vi "Fetch Multiple Record Single Channel (U64).vi"(5 "FIFO Type":enum16{"FPGA to Host FIFO (U64)", "Generic"}(ring), 7 "Timeout (s)":i32=5, 8 "error in":errorcluster, 10 "Records to Fetch":i32, 11 "FPGA VI Reference In":refnum<k20>) -> (0 "error out":errorcluster, 2 "Acquired Data":u64[](array[numeric]), 3 "FPGA VI Reference Out":refnum<k20>, 4 "Elements Remaining":u32)   [LabVIEW 2011]
uses:
  <userlib>/FlexRIO Host Library/FlexRIO Host API/Acquire/Fetch/Fetch Acquired Data (U64).vi
  <vilib>/Utility/error.llb/Error Cluster From Error Code.vi
  <vilib>/rvi/errors/niLvFpgaAdjustHostInterfaceError.vi
  <vilib>/rvi/interface/nirviReadWriteControl/nirviReadWriteControl.xnode
  NiFpgaLv.dll
  <vilib>/rvi/interface/Simulation/niFpgaSimulationCallBeginRW.vi
  <userlib>/FlexRIO Host Library/FlexRIO Host Library (User).lvlib
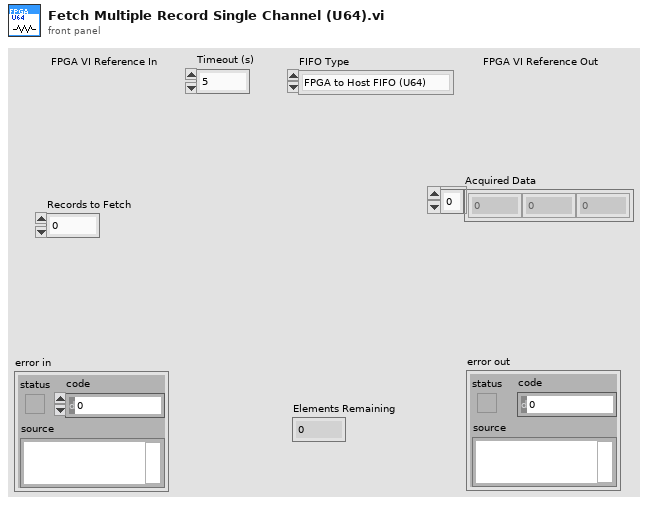
[diagram p1: front panel]
types:
  T1 = cluster{"Load Record Parameters?":bool, "Pre Trigger Samples":u16, "Samples per Record":u16, "Trigger Hold Off":u16, "Record Count":u16}
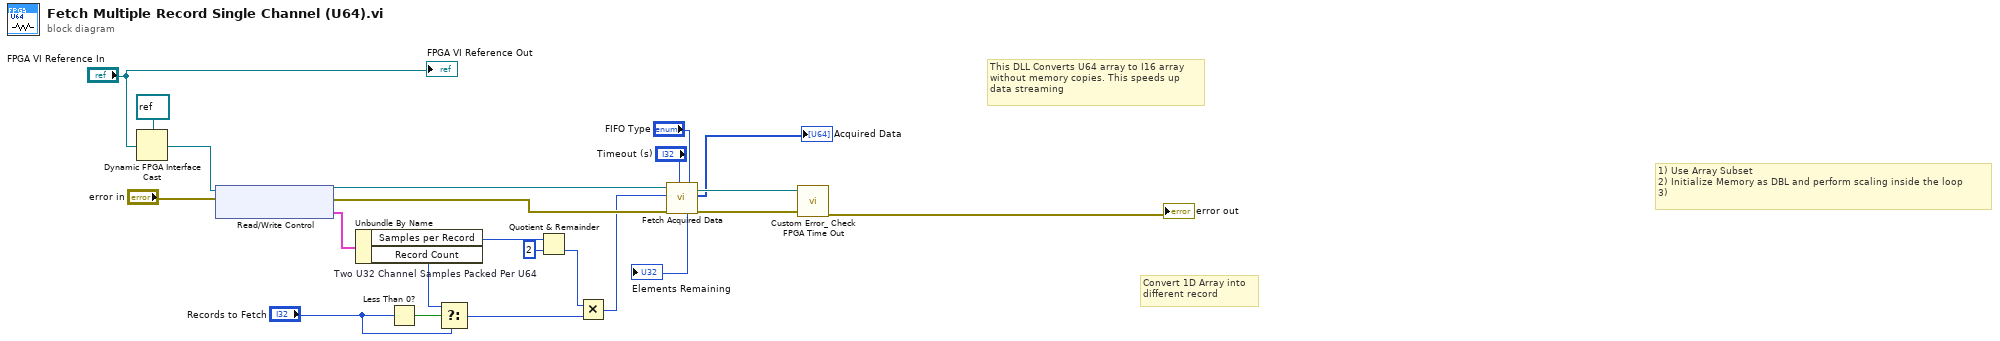
[diagram p0: block diagram]
diagram:
  w5 = u16 2  # Two U32 Channel Samples Packed Per U64
  # "This DLL Converts U64 array to I16 array \nwithout memory copies. This speeds up \ndata streaming"
  # "Convert 1D Array into\ndifferent record"
  # "1) Use Array Subset\n2) Initialize Memory as DBL and perform scaling inside the loop\n3)"
  n1 = Dynamic FPGA Interface Cast(Session In=refnum<k20> refnum ("Type"), Type="FPGA VI Reference In") -> (Session Out=w19:refnum<k20>)
  n2 = xnode "Read/Write Control"("FPGA VI Reference In"=w19, "error in"="error in") -> ("FPGA VI Reference Out"=w14:refnum<k20>, "error out"=w13:errorcluster, "Record Parameters"=w18:T1)
  n3 = Unbundle By Name(w18) -> ("Samples per Record"=w6:u16, "Record Count"=w16:u16)
  n4 = Less Than 0?(x="Records to Fetch") -> (x < 0?=w17:bool)
  n5 = Select(t=w16, s=w17, f="Records to Fetch") -> (s? t:f=w2:i32)
  n6 = Quotient & Remainder(x=w6, y=w5) -> (floor(x/y)=w3:u16)  [unwired: 1 out]
  n7 = Multiply(x=w3, y=w2) -> (x*y=w7:i32)
  n8 = call-poly <userlib>:"Fetch Acquired Data.vi"("FIFO Type"="FIFO Type", "Timeout (s)"="Timeout (s)", "error out"=w13, "Samples"=w7, "FPGA Reference In"=w14) -> ("error out"=w8:errorcluster, "Data"=→"Acquired Data":u64[], "FPGA Reference Out"=w9:refnum<k20>, "Elements Remaining"=→"Elements Remaining":u32)  [unwired: 3 in]
  n9 = call <userlib>:"Custom Error_ Check FPGA Time Out.vi"("error in"=w8, "FPGA VI Reference In"=w9) -> ("error out"=→"error out":errorcluster)  [unwired: 8 in, 1 out]
  "FPGA VI Reference Out" <- "FPGA VI Reference In"
